vi "Global GUI Variable.vi"() -> ()   [LabVIEW 2014]
panel:
  out "target indicators":string
  out "Temp Diff":string
  out "GUI status":string
  out "Thermometer":sgl
  out "target":string
  out "stop  button2":bool
  out "heater status":bool
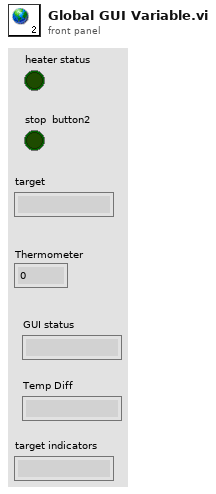
[diagram p1: front panel]
diagram:
